vi "Sensor_Values.vi"() -> ()   [LabVIEW 2019]
panel:
  out "Climb_Bottom_Limit":bool
  out "Climb_Top_Limit":bool
  in  "Elevator_Left_Position(Native)":dbl
  in  "Elevator_Right_Position(Native)":dbl
  in  "Control_Panel_Velocity(RPM)":dbl
  in  "Control_Panel_Position":dbl
  in  "Turret_Velocity(RPM)":dbl
  in  "Turret_Position":dbl
  in  "Magazine_Velocity(RPM)":dbl
  in  "Magazine_Position":dbl
  in  "Flywheel_Right_Velocity(RPM)":dbl
  in  "Flywheel_Left_Velocity(RPM)":dbl
  in  "Right_Drive_Position":dbl
  in  "Left_Drive_Position":dbl
  in  "Right_Drive_Velocity(RPM)":dbl
  in  "Left_Drive_Velocity(RPM)":dbl
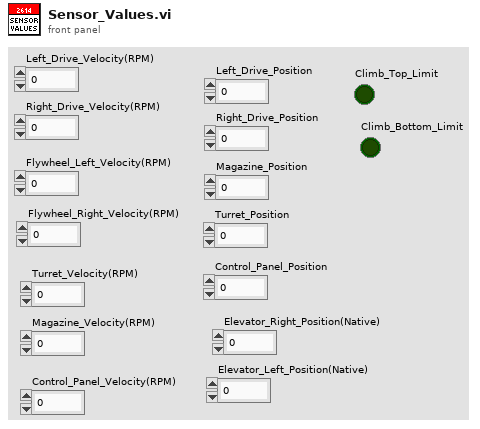
[diagram p1: front panel]
diagram:
